vi "Both Mic Data seperately acquired.vi"() -> ()   [LabVIEW 2021]
uses:
  <vilib>/ptbypt/NI_PtbyPt.lvlib
panel:
  in  "rate":dbl=51200.0
  in  "number of samples":i32=10000
  out "Waveform Chart 2":dynamicdata(graph)
  out "Waveform Chart":dynamicdata(graph)
  in  "stop (F)":bool
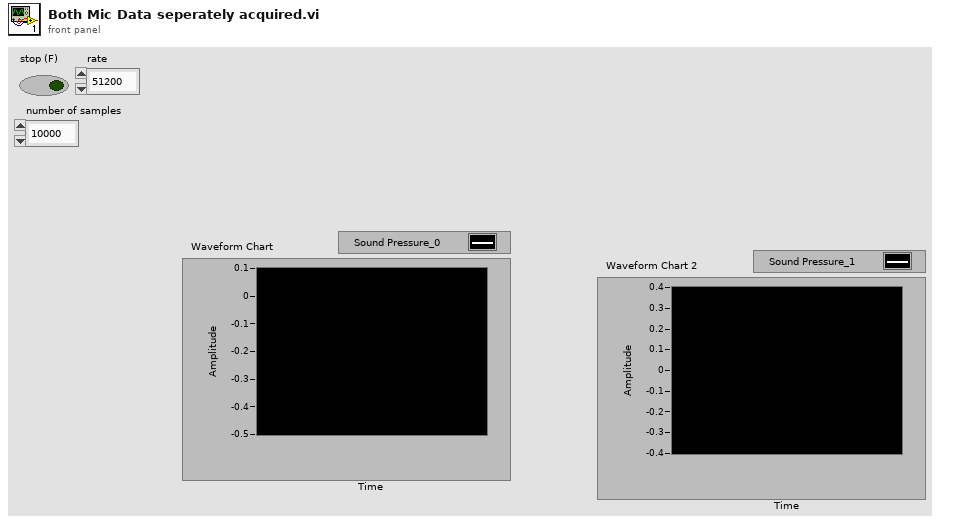
[diagram p1: front panel]
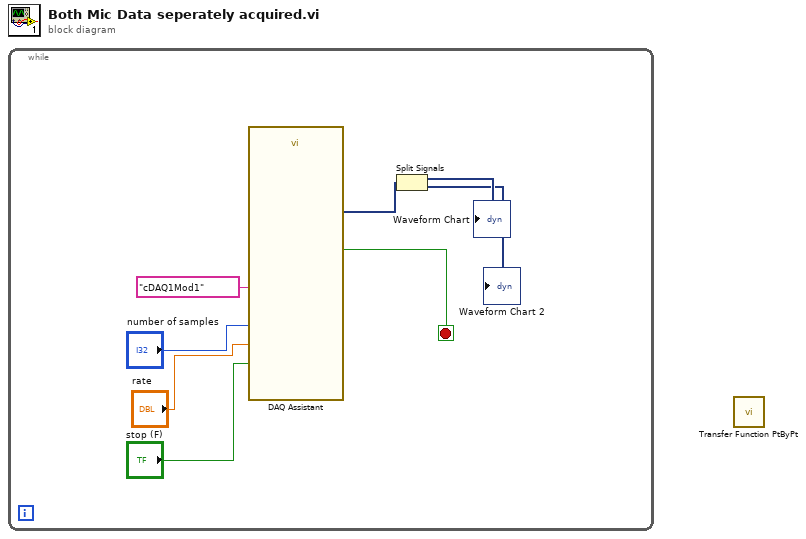
[diagram p0: block diagram]
diagram:
  n1 = while {
    stop <- w7 stop-if-true
    n2 = call "DAQ Assistant"("rate"="rate", "number of samples"="number of samples", "stop (F)"="stop (F)", "device name"=tag "cDAQ1Mod1") -> ("data"=w4:dynamicdata, "stopped"=w7:bool)  [unwired: 12 in, 2 out]
    n3 = Split Signals(w4) -> (→"Waveform Chart":dynamicdata, →"Waveform Chart 2":dynamicdata)  [unwired: 2 in]
  }
  n4 = call <vilib>:"Transfer Function PtByPt.vi"() -> ()  [unwired: 5 in, 4 out]
